vi "Configure Trigger Sweep Signal.vi"(6 "Delay (0 s)":dbl, 7 "Trigger Level (1: Low)":i32(ring)=1 items=["High", "Low"], 8 "error in (no error)":errorcluster, 9 "Trigger Scope (0: All)":i32(ring) items=["All", "Current"], 10 "Trigger Source (0: Immediate)":i32(ring) items=["Immediate", "External", "Manual"], 11 "VISA resource name":refnum<visa-resource-name>) -> (0 "error out":errorcluster, 3 "VISA resource name out":refnum<visa-resource-name>)   [LabVIEW 2018, in "Keysight PNA Series.lvlib"]
doc: "Configures the trigger sweep signal."
uses:
  Keysight PNA Series.lvlib
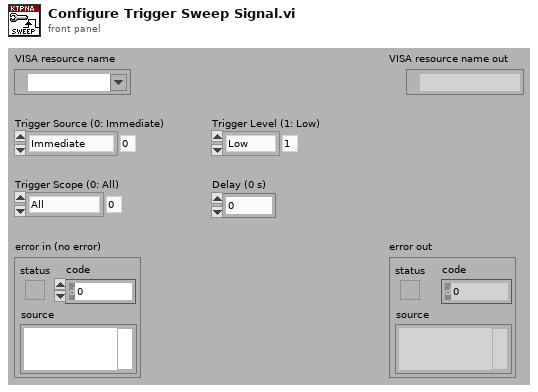
[diagram p1: front panel]
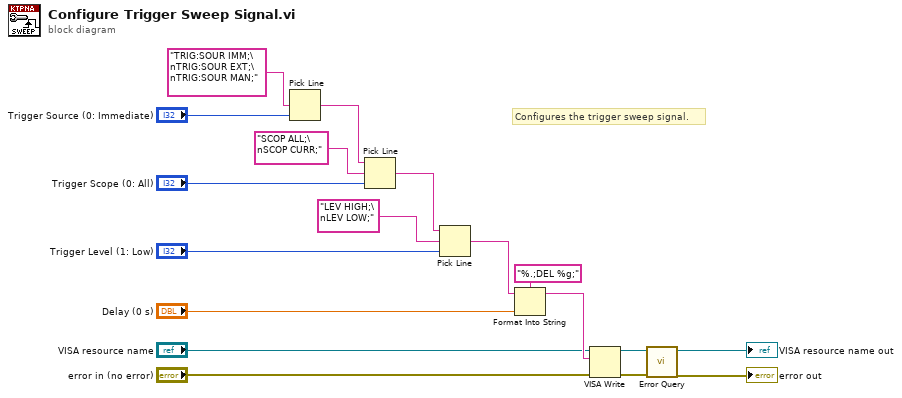
[diagram p0: block diagram]
diagram:
  # "Configures the trigger sweep signal."
  n1 = Pick Line(multi-line string="TRIG:SOUR IMM;\nTRIG:SOUR EXT;\nTRIG:SOUR MAN;", line index="Trigger Source (0: Immediate)") -> (output string=w14:string)  [unwired: 1 in]
  n2 = Pick Line(string ("")=w14, multi-line string="SCOP ALL;\nSCOP CURR;", line index="Trigger Scope (0: All)") -> (output string=w11:string)
  n3 = Pick Line(string ("")=w11, multi-line string="LEV HIGH;\nLEV LOW;", line index="Trigger Level (1: Low)") -> (output string=w10:string)
  n4 = Format Into String(format string="%.;DEL %g;", initial string=w10, "Delay (0 s)") -> (resulting string=w7:string)  [unwired: 1 in, 1 out]
  n5 = VISA Write(VISA resource name="VISA resource name", write buffer=w7, error in (no error)="error in (no error)") -> (VISA resource name out=w4:refnum<visa-resource-name>, error out=w3:errorcluster)  [unwired: 1 out]
  n6 = call "Error Query.vi"("error in (no error)"=w3, "VISA resource name"=w4) -> ("error out"=→"error out":errorcluster, "VISA resource name out"=→"VISA resource name out":refnum<visa-resource-name>)  [unwired: 6 in, 2 out]
